vi "Project Items - Keep VIs.vi"(8 "Error In":errorcluster, 11 "Project Items":refnum<vi>[](array[refnum])) -> (0 "Error Out":errorcluster, 3 "Project Items (VIs)":refnum<vi>[](array[refnum]))   [LabVIEW 2022 SP3]
doc: "<add documentation here>"
panel:
  # "Development\nControls or indicators that are useful for development or testing, but which are not outputs of the VI."
  # "Input\nInputs to the VI"
  # "Output\nOutputs of the VI"
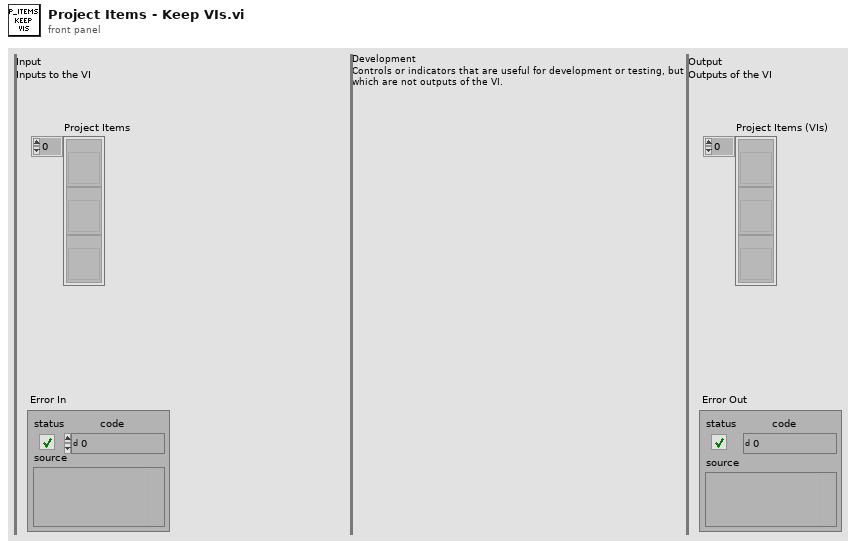
[diagram p1: front panel]
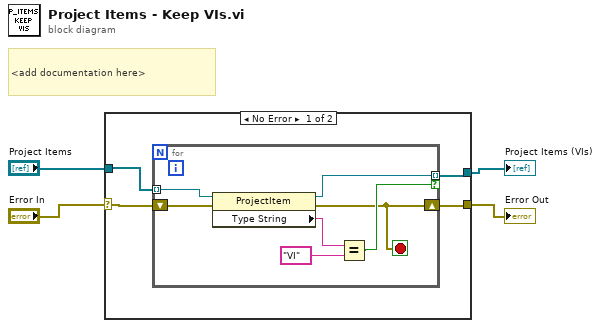
[diagram p0: block diagram]
diagram:
  # "<add documentation here>"
  n1 = case shown="No Error" "Error In" {
    selector: "Error In" -> [w8 w16]
    tunnel: [w6 w16] -> w3
    tunnel: "Project Items" -> [w7 _]
    tunnel: [w5 _] -> w1
    frame No Error {
      n2 = for {
        tunnel: w7 -> [w15] mode=indexing
        shift-right: [w9] -> w6
        shift-left: w8 -> [w14]
        tunnel: [w11] -> w5 mode=indexing if=w10
        stop <- w9 stop-if-true
        n3 = property class="ProjectItem"(reference=w15, error in=w14) -> (reference out=w11:refnum<vi>, error out=w9:errorcluster, "Type String"=w13:string)
        n4 = Equal?(x=w13, y="VI") -> (x = y?=w10:bool)
      }
    }
    frame Error {
    }
  }
  "Error Out" <- w3
  "Project Items (VIs)" <- w1
